vi "Wait For Deploy.vi"(11 "RTTarget in":refnum<class "RTTarget.lvclass">) -> (0 "deployed":bool, 3 "RTTarget out":refnum<class "RTTarget.lvclass">)   [LabVIEW 2020, in "NI_TargetHelper.lvlib" / "RTTarget.lvclass"]
uses:
  <vilib>/TargetSupport/NI_TargetHelper/RTTarget/RTTarget.lvclass
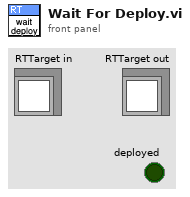
[diagram p1: front panel]
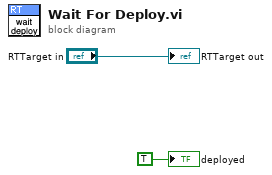
[diagram p0: block diagram]
diagram:
  "RTTarget out" <- "RTTarget in"
  "deployed" <- TRUE ("deployed")
